vi "ObtainRequestEvents.vi"(8 "error in (no error)":errorcluster, 10 "CreateNew (F)":bool) -> (0 "error out":errorcluster, 2 "clRequestEvents":T1)   [LabVIEW 2018, in "SensorShared.lvlib"]
uses:
  SensorShared.lvlib
  clRequestEvents.ctl
  clEventType.ctl
panel:
  # "If you want to add other Request Events, open this typedef, copy an existing event and rename it to your Request name.\n\nNext create a typedef for the  data and put it into PublicAPI/Arguments/Requests\n\nNext, add an event handler loop event case in Main.vi to handle the new request event\n\nMost likely, each request will also require the creation of a new Queued Message Handler loop case in Main.VI"
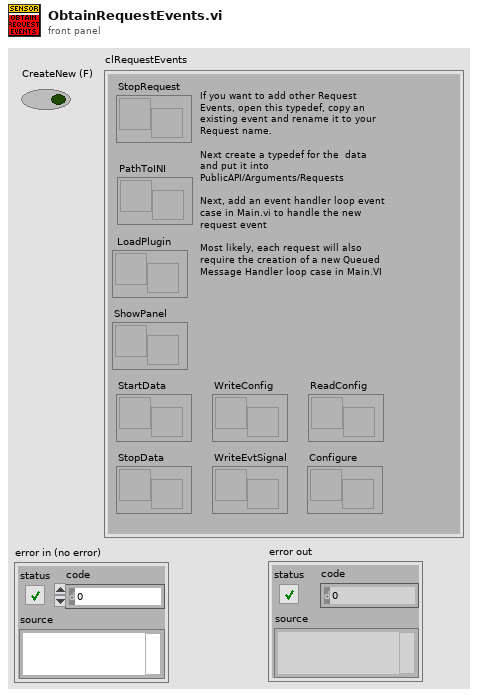
[diagram p1: front panel]
types:
  T1 = typedef "SensorShared.lvlib/clRequestEvents.ctl" = cluster{"StopRequest":refnum<user-event>, "PathToINI":refnum<user-event>, " LoadPlugin":refnum<user-event>, "ShowPanel":refnum<user-event>, "StartData":refnum<user-event>, "StopData":refnum<user-event>, "WriteConfig":refnum<user-event>, "ReadConfig":refnum<user-event>, "WriteEvtSignal":refnum<user-event>, "Configure":refnum<user-event>}
  T2 = typedef "SensorModule.lvlib/clRequestEvents.ctl" = cluster{"StopRequest":refnum<user-event>, "PathToINI":refnum<user-event>, " LoadPlugin":refnum<user-event>, "ShowPanel":refnum<user-event>, "StartData":refnum<user-event>, "StopData":refnum<user-event>, "WriteConfig":refnum<user-event>, "ReadConfig":refnum<user-event>, "WriteEvtSignal":refnum<user-event>, "Configure":refnum<user-event>}
  T3 = typedef "SensorShared.lvlib/clEventType.ctl" = cluster{"ModuleID":i32, "Data":variant}
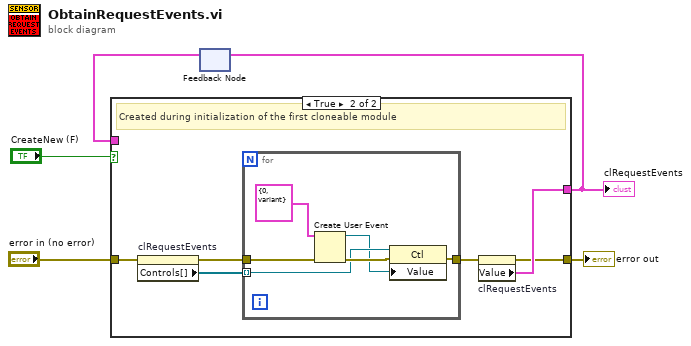
[diagram p0: block diagram]
diagram:
  n1 = feedback #1() -> (w3:T2)  [unwired: 1 in]
  n2 = case shown="True" "CreateNew (F)" {
    tunnel: "error in (no error)" -> [w7 w13]
    tunnel: w3 -> [w6 _]
    tunnel: [w7 w8] -> w2
    tunnel: [w6 w10] -> w1
    frame False {
    }
    frame True {
      # "Created during initialization of the first cloneable module"
      n3 = property on="clRequestEvents" class="Clust (strict)"(error in=w13) -> (error out=w11:errorcluster, "Controls[]"=w12:refnum<vi>[])  [unwired: 1 in, 1 out]
      n4 = for {
        tunnel: w12 -> [w15] mode=indexing
        tunnel: w11 -> [w18]
        tunnel: [w16] -> w9
        n5 = Create User Event(user event datatype=T3 {"ModuleID"=0, "Data"=variant} ("clEventType"), error in=w18) -> (user event=w14:refnum<user-event>, error out=w17:errorcluster)
        n6 = property on="Property Node" class="Ctl"(reference=w15, error in=w17, "Value"=w14) -> (error out=w16:errorcluster)  [unwired: 1 out]
      }
      n7 = property on="clRequestEvents" class="Clust (strict)"(error in=w9) -> (error out=w8:errorcluster, "Value"=w10:T2)  [unwired: 1 in, 1 out]
    }
  }
  "error out" <- w2
  "clRequestEvents" <- w1
  n8 = feedback-in #1(w1) -> ()
